vi "RT_stagectrl_readIFO_Oct.vi"() -> ()   [LabVIEW 2019]
uses:
  <vilib>/Platform/TimedLoop/XDataNode/timing_clust.ctl
  <vilib>/Platform/TimedLoop/XDataNode/nitl_modes.ctl
  <vilib>/Platform/TimedLoop/XDataNode/wakeup.ctl
  <vilib>/Analysis/baseanly.llb/Mean (DBL).vi
  <vilib>/FPGAPlugInAG/myRIO-1900/niLvFpga_Open_myRIO-1900.vi
  <vilib>/rvi/interface/common/dynamic/niFpgaDynamicAddResources.vi
  <vilib>/Utility/error.llb/Error Cluster From Error Code.vi
  <vilib>/rvi/errors/niLvFpgaAdjustHostInterfaceError.vi
  <vilib>/FPGAPlugInAG/Dynamic/niLvFpga_Close_Dynamic.vi
  <vilib>/rvi/interface/nirviOpenFPGA/nirviOpenFPGA.xnode
  FPGA Bitfiles/studentchallenge_FPGATarget_FPGA1RADC1WDAC2A_GeAN6BgpSew.lvbitx
  <vilib>/rvi/interface/nirviReadWriteControl/nirviReadWriteControl.xnode
  <vilib>/platform/TimedLoop/XDataNode/XDataNode.xnode
  <vilib>/rvi/interface/nirviCloseFPGA/nirviCloseFPGA.xnode
  NiFpgaLv.dll
  <vilib>/rvi/interface/Simulation/niFpgaSimulationCallBeginRW.vi
  <vilib>/Platform/TimedLoop/XDataNode/XDNodeRunTimeDep.lvlib
  <vilib>/Analysis/NI_AALBase.lvlib
panel:
  out "Z (um)":dbl(graph)=-1075.0316368535157
  in  "Stop":bool=TRUE
  in  "P":dbl=1.0
  in  "I":dbl=0.003
  in  "D":dbl
  out "Control voltage":dbl=-10.0 format="%#_3f"
  out "Encoder position (mm)":dbl=-1.05 format="%#_4f"
  out "late?":bool
  in  "Ramp ON":bool
  out "Mid-travel (mm)":dbl format="%#_3f"
  out "?":dynamicdata(graph)=[{"t0"=timestamp(2082851436.547542 s since 1904-01-01), "dt"=1.0, "Y"=[0.0]}, {"t0"=timestamp(2082851436.547623 s since 1904-01-01), "dt"=1.0, "Y"=[-1.05]}]
  in  "Stage loop time (us)":i64=2000
  in  "Velocity (mm/s)":dbl=0.3 format="%#_3g"
  in  "Ramp Vpp (mm)":dbl=2.0 format="%#_13g"
  out "Vp":dbl=1.05
  out "Vi":dbl=10.0
  out "Vd":dbl
  out "Lissajou":cluster{"X":dbl[], "Y":dbl[]}[](graph)
  out "?":dynamicdata(graph)=[{"t0"=timestamp(2082851436.54781 s since 1904-01-01), "dt"=1.0, "Y"=[2.36669921875]}, {"t0"=timestamp(2082851436.547639 s since 1904-01-01), "dt"=1.0, "Y"=[2.148193359375]}]
  in  "IFO plot loop time (us)":i64=1000
  out "late?":bool
  out "FWD limit flag":bool
  out "REV lim (mm)":dbl=-2.7246875 format="%#_5f"
  out "FWD lim (mm)":dbl=10.833828125 format="%#_5f"
  out "Voltage":dbl=3.5999999999999956
  out "REV limit flag":bool=TRUE
  out "Position (mm)":dbl(slide)=-2.7246875 scale=-10.0..10.0
  out "Vfwd":dbl=0.2499999999999999
  out "Vrev":dbl=-3.5999999999999956
  out "ENC0":i32=70
  out "Enc res (mm)":dbl=7.8125e-05
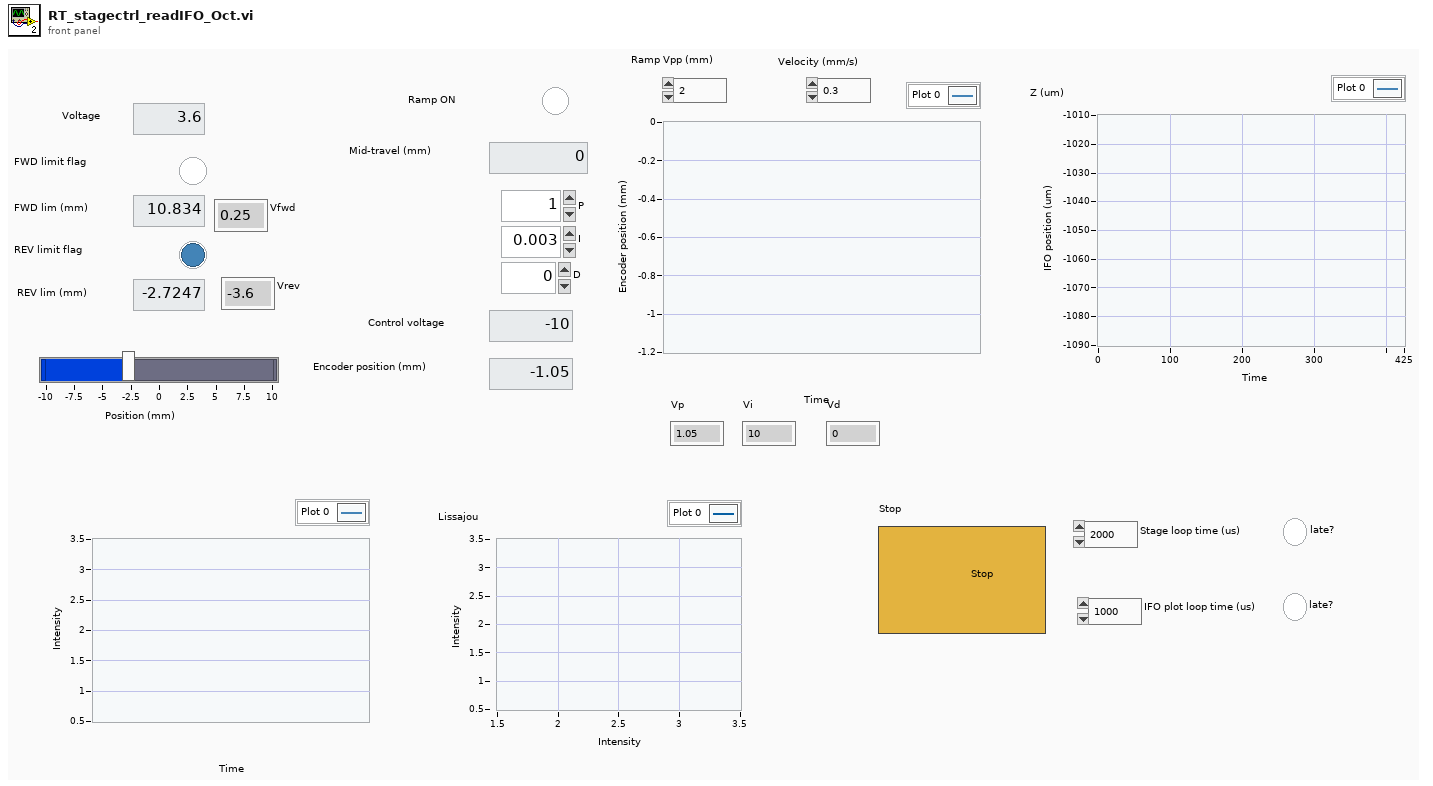
[diagram p1: front panel]
types:
  T1 = typedef "XDNodeRunTimeDep.lvlib/timing_clust.ctl" = cluster{"Expected End [f-1]":u64, "Actual End [f-1]":u64, "Finished Late? [f-1]":bool, "Expected End [i-1]":u64, "Actual End [i-1]":u64, "Finished Late? [i-1]":bool, "Expected Start [i]":u64, "Actual Start [i]":u64, "Expected Start [f]":u64, "Actual Start [f]":u64, "Source Name":string, "Structure Name":string, "Period":i64, "Deadline":i64, "Offset":i64, "Start":i64, "Priority":i32, "Timeout":i32, "Mode":T2, "Wakeup Reason":T3, "Error":errorcluster, "Source Type":string, "Secondary Source Type":string, "Global End Time":u64, "Global Start Time":u64, "Frame Duration":u64, "Iteration Duration":u64, "Assigned CPU":i32, "I/O Scan Engine Mode":u32}
  T2 = typedef "XDNodeRunTimeDep.lvlib/nitl_modes.ctl" = enum32{"No Change", "Process missed periods, maintain original phase", "Discard missed periods, maintain original phase", "Process missed periods, ignore original phase", "Discard missed periods, ignore original phase"}
  T3 = typedef "XDNodeRunTimeDep.lvlib/wakeup.ctl" = enum32{"Normal", "Aborted", "Asynchronous wakeup", "Timing source error", "Timed loop error", "Timeout"}
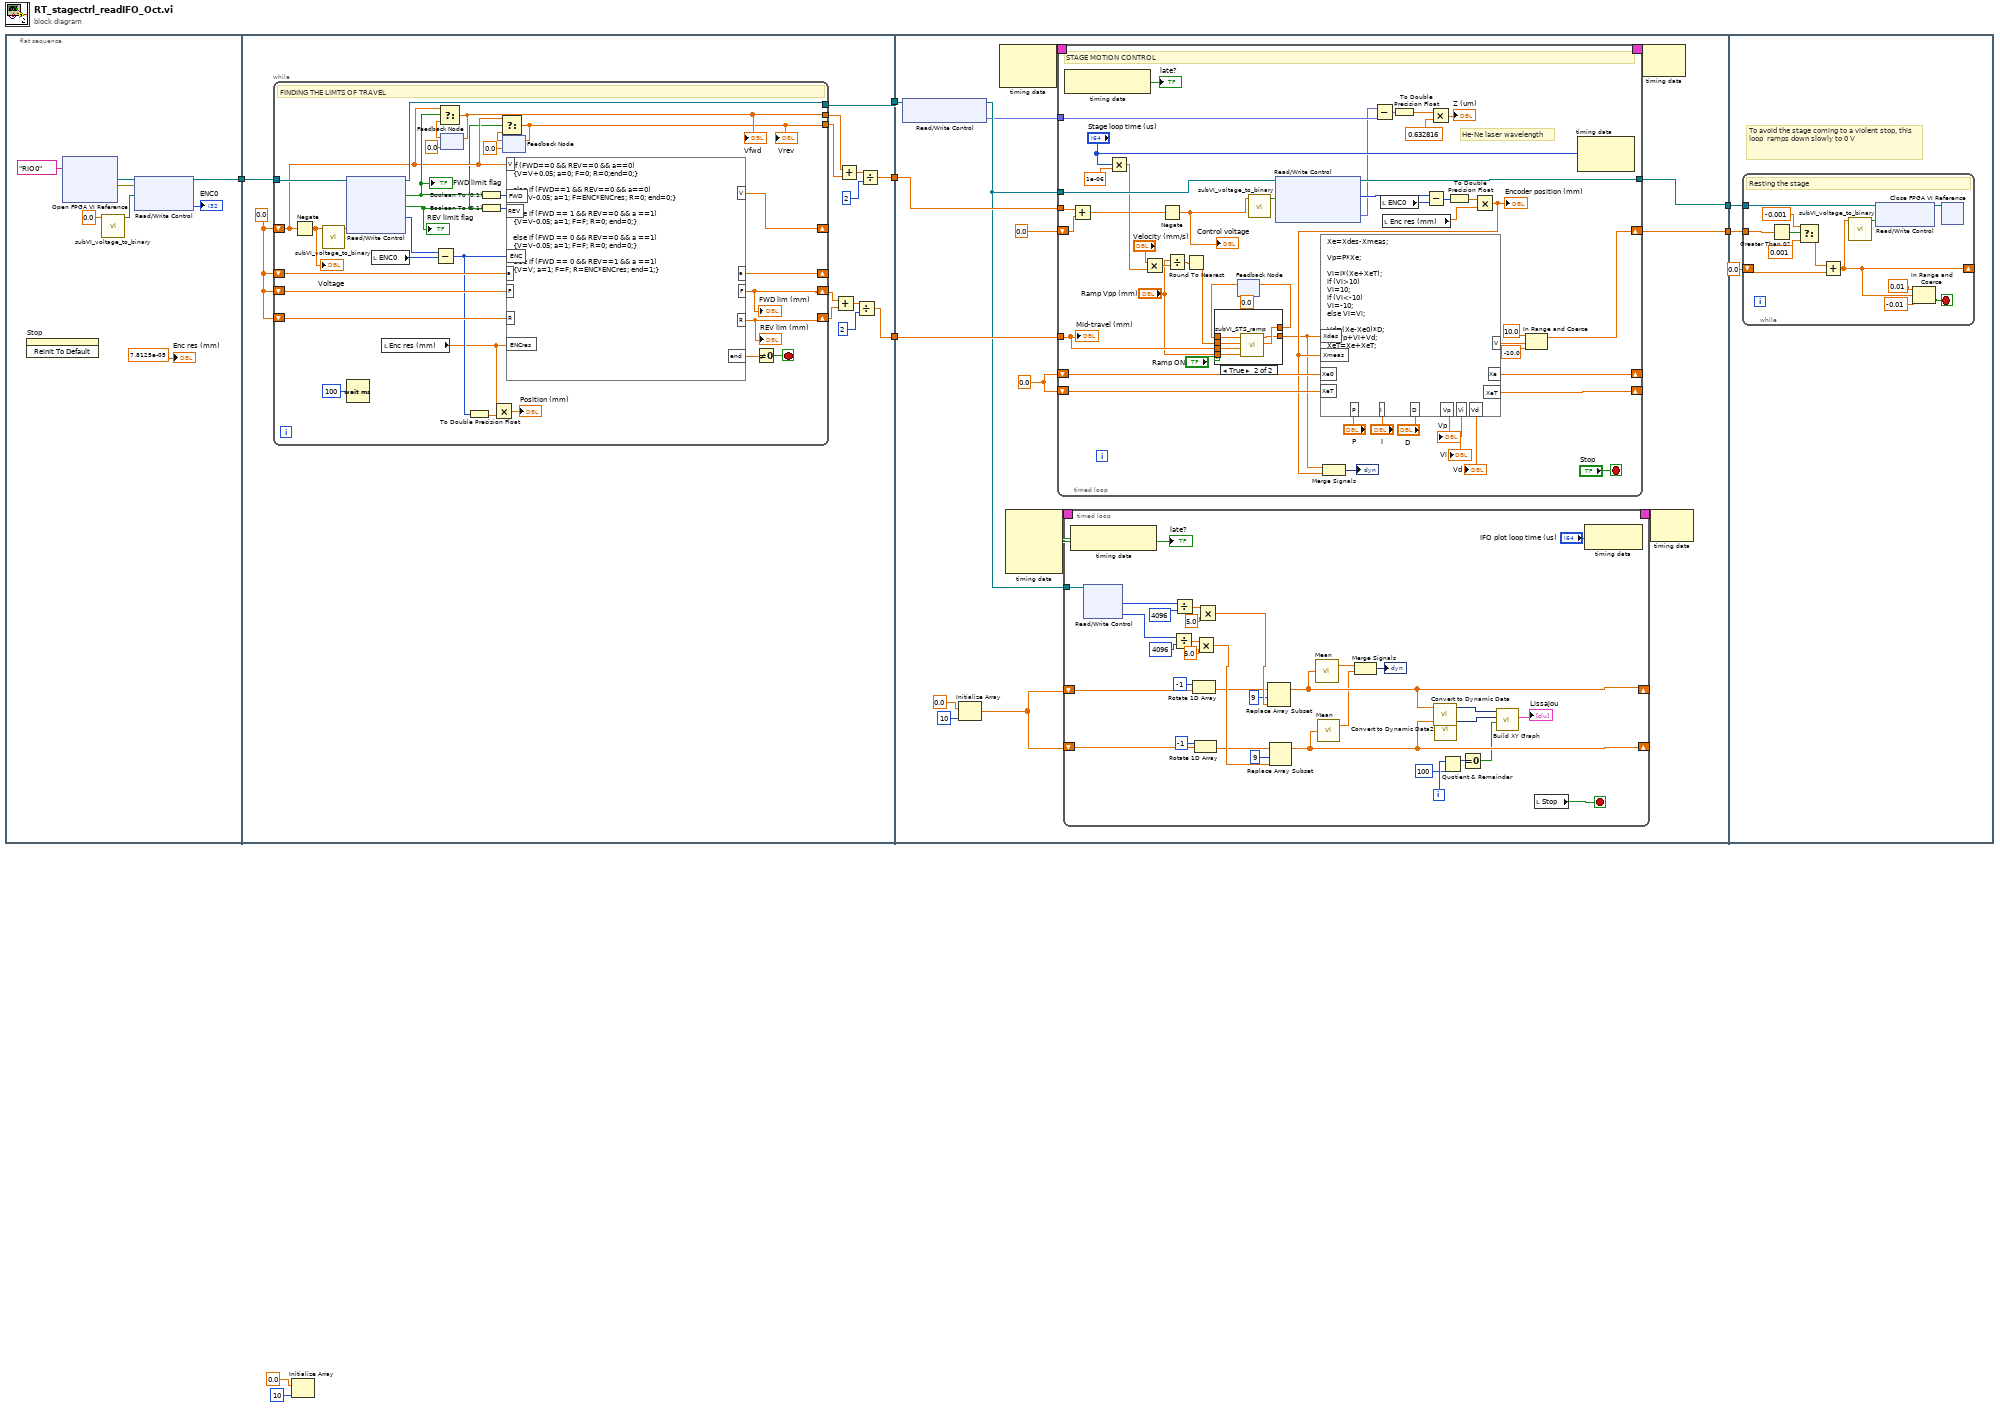
[diagram p0: block diagram]
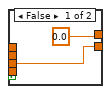
[diagram p2: hidden frame]
diagram:
  n1 = flat-sequence {
    tunnel: [w16] -> w8
    tunnel: w8 -> [w27]
    tunnel: [w29] -> w7
    tunnel: [w17] -> w6
    tunnel: [w28] -> w5
    tunnel: [w62] -> w4
    tunnel: w7 -> [w74]
    tunnel: w6 -> [w64]
    tunnel: [w73] -> w3
    tunnel: w5 -> [w65]
    tunnel: w4 -> [w185]
    tunnel: w3 -> [w184]
    frame #0 {
      n2 = invoke on="Stop" class="Bool (strict)" method="Reinit To Default"() -> ()  [unwired: 3 in, 3 out]
      n3 = xnode "Open FPGA VI Reference"("resource name"=tag "RIO0") -> ("FPGA VI Reference Out"=w9:refnum<k20>, "error out"=w14:errorcluster)  [unwired: 1 in]
      n4 = call "subVI_voltage_to_binary.vi"("voltage"=0.0) -> ("binary"=w12:bool[])  [unwired: 10 in]
      n5 = xnode "Read/Write Control"("FPGA VI Reference In"=w9, "error in"=w14, "DAC 1 write"=w12) -> ("FPGA VI Reference Out"=w16:refnum<k20>, "Encoder A"=→"ENC0":i32)  [unwired: 1 out]
      "Enc res (mm)" <- 7.8125e-05 ("y")
    }
    frame #1 {
      w22 = 0.0 ("V")
      n6 = while {
        shift-right: [w44] -> _
        shift-left: w22 -> [w33]
        shift-right: [w60] -> _
        shift-left: w22 -> [w59]
        shift-right: [w45] -> w24
        shift-left: w22 -> [w53]
        shift-right: [w46] -> w23
        shift-left: w22 -> [w52]
        tunnel: w27 -> [w50]
        tunnel: [w48] -> w17
        tunnel: [w31] -> w20
        tunnel: [w30] -> w19
        stop <- w55 stop-if-true
        # "FINDING THE LIMTS OF TRAVEL"
        n7 = Negate(x=w33) -> (-x=w39:dbl)
        "Voltage" <- w39
        n8 = call "subVI_voltage_to_binary.vi"("voltage"=w39) -> ("binary"=w51:bool[])  [unwired: 10 in]
        n9 = xnode "Read/Write Control"("FPGA VI Reference In"=w50, "DAC 1 write"=w51) -> ("FPGA VI Reference Out"=w48:refnum<k20>, "YFWD"=w38:bool, "YREV"=w32:bool, "Encoder A"=w54:i32)  [unwired: 1 in, 1 out]
        "FWD limit flag" <- w38
        "REV limit flag" <- w32
        n10 = Wait (ms)(milliseconds to wait=u32 100) -> ()  [unwired: 1 out]
        n11 = local read "ENC0"() -> (w49:i32)
        n12 = local read "Enc res (mm)"() -> (w41:dbl)
        n13 = Subtract(x=w54, y=w49) -> (x-y=w43:i32)
        n14 = feedback #1(0.0 ("V")) -> (w37:dbl)
        n15 = Select(t=w33, s=w38, f=w37) -> (s? t:f=w31:dbl)
        "Vfwd" <- w31
        n16 = feedback-in #1(w31) -> ()
        n17 = To Double Precision Float(number=w43) -> (double precision float=w40:dbl)
        n18 = Boolean To (0,1)(Boolean=w38) -> (0, 1=w58:i16)
        n19 = Boolean To (0,1)(Boolean=w32) -> (0, 1=w57:i16)
        n20 = Multiply(x=w41, y=w40) -> (x*y=→"Position (mm)":dbl)
        n21 = feedback #2(0.0 ("V")) -> (w35:dbl)
        n22 = Select(t=w33, s=w32, f=w35) -> (s? t:f=w30:dbl)
        "Vrev" <- w30
        n23 = feedback-in #2(w30) -> ()
        n24 = formula code="if (FWD==0 && REV==0 && a==0)\n{V=V+0.05; a=0; F=0; R=0;end=0;}\n\nelse if (FWD==1 && REV==0 && a==0)\n{V=V-0.05; a=1; F=ENC*ENCres; R=0; end=0;}\n\nelse if (FWD == 1 && REV==0 && a ==1)\n{V=V-0.05; a=1; F=F; R=0; end=0;}\n\nelse if (FWD == 0 && REV==0 && a ==1)\n{V=V-0.05; a=1; F=F; R=0; end=0;}\n\nelse if (FWD == 0 && REV==1 && a ==1)\n{V=V; a=1; F=F; R=ENC*ENCres; end=1;}"("FWD"=w58, "REV"=w57, "a"=w59, "ENC"=w43, "F"=w53, "R"=w52, "V"=w33, "ENCres"=w41) -> ("V"=w44:dbl, "a"=w60:dbl, "end"=w56:dbl, "F"=w45:dbl, "R"=w46:dbl)
        "REV lim (mm)" <- w46
        "FWD lim (mm)" <- w45
        n25 = Not Equal To 0?(x=w56) -> (x != 0?=w55:bool)
      }
      n26 = Add(x=w24, y=w23) -> (x+y=w26:dbl)
      n27 = Add(x=w20, y=w19) -> (x+y=w18:dbl)
      n28 = Divide(x=w26, y=2) -> (x/y=w29:dbl)
      n29 = Divide(x=w18, y=2) -> (x/y=w28:dbl)
    }
    frame #2 {
      w67 = 0.0 ("Xe")
      n30 = xnode "Read/Write Control"("FPGA VI Reference In"=w64) -> ("FPGA VI Reference Out"=w63:refnum<k20>, "unwrapped phase"=w61:fxp<+/-,47,33>)  [unwired: 1 in, 1 out]
      n31 = Initialize Array(0.0 ("element"), 10 ("dimension size")) -> (w68:dbl[])
      n32 = node-c288() -> (w76:T1)  [unwired: 2 in]
      n33 = node-c288() -> (w72:T1)  [unwired: 4 in]
      n34 = timed-loop {
        timing: w76 -> [_]
        timing-out: [_] -> w75
        tunnel: [w163] -> w62
        tunnel: w74 -> [w133]
        shift-right: [w148] -> w73
        shift-left: 0.0 ("upper limit") -> [w127]
        tunnel: w63 -> [w161]
        shift-right: [w156] -> _
        shift-left: w67 -> [w155]
        shift-right: [w154] -> _
        shift-left: w67 -> [w153]
        tunnel: w65 -> [w126]
        tunnel: w61 -> [w120]
        stop <- "Stop" stop-if-true
        # "He-Ne laser wavelength"
        # "STAGE MOTION CONTROL"
        n35 = node-c288() -> (→"late?":bool)  [unwired: 1 in]
        n36 = Add(x=w126, y=w127) -> (x+y=w124:dbl)
        n37 = Multiply(x="Stage loop time (us)", y=1e-06) -> (x*y=w141:dbl)
        n38 = Multiply(x="Velocity (mm/s)", y=w141) -> (x*y=w144:dbl)
        n39 = Negate(x=w124) -> (-x=w125:dbl)
        "Control voltage" <- w125
        n40 = Divide(x="Ramp Vpp (mm)", y=w144) -> (x/y=w139:dbl)
        n41 = Round To Nearest(number=w139) -> (nearest integer value=w134:dbl)
        n42 = feedback #3(0.0 ("n1")) -> (w136:dbl)
        n43 = case shown="True" "Ramp ON" {
          tunnel: w136 -> [_ w175]
          tunnel: [0.0 ("n1") w174] -> w135
          tunnel: w134 -> [_ w173]
          tunnel: w133 -> [w169 w172]
          tunnel: [w169 w171] -> w131
          tunnel: "Ramp Vpp (mm)" -> [_ w170]
          frame False {
          }
          frame True {
            n44 = call "subVI_STS_ramp.vi"("Ramp Vpp"=w170, "Ramp offset"=w172, "Ramp datapoints"=w173, "n"=w175) -> ("n1"=w174:dbl, "Ramp out"=w171:dbl)  [unwired: 6 in]
          }
        }
        n45 = feedback-in #3(w135) -> ()
        n46 = call "subVI_voltage_to_binary.vi"("voltage"=w125) -> ("binary"=w164:bool[])  [unwired: 10 in]
        n47 = xnode "Read/Write Control"("FPGA VI Reference In"=w161, "DAC 1 write"=w164) -> ("FPGA VI Reference Out"=w163:refnum<k20>, "Encoder A"=w165:i32, "unwrapped phase"=w119:fxp<+/-,47,33>)  [unwired: 1 in, 1 out]
        n48 = Subtract(x=w119, y=w120) -> (x-y=w121:fxp<+/-,48,34>)
        n49 = local read "ENC0"() -> (w162:i32)
        n50 = local read "Enc res (mm)"() -> (w145:dbl)
        n51 = To Double Precision Float(number=w121) -> (double precision float=w123:dbl)
        n52 = Subtract(x=w165, y=w162) -> (x-y=w166:i32)
        n53 = Multiply(x=w123, y=0.632816) -> (x*y=→"Z (um)":dbl)
        n54 = To Double Precision Float(number=w166) -> (double precision float=w167:dbl)
        n55 = Multiply(x=w167, y=w145) -> (x*y=w146:dbl)
        "Encoder position (mm)" <- w146
        n56 = formula code="Xe=Xdes-Xmeas;\n\nVp=P*Xe;\n\nVi=I*(Xe+XeT);\nif (Vi>10)\nVi=10;\nif (Vi<-10)\nVi=-10;\nelse Vi=Vi;\n\nVd=(Xe-Xe0)*D;\nV=Vp+Vi+Vd;\nXeT=Xe+XeT;"("Xdes"=w131, "Xmeas"=w146, "Xe0"=w155, "XeT"=w153, "P"="P", "I"="I", "D"="D") -> ("Xe"=w156:dbl, "V"=w157:dbl, "XeT"=w154:dbl, "Vp"=→"Vp":dbl, "Vi"=→"Vi":dbl, "Vd"=→"Vd":dbl)
        n57 = Merge Signals(w131, w146) -> (→"?":dynamicdata)
        n58 = In Range and Coerce(upper limit=10.0, x=w157, lower limit=-10.0) -> (coerced(x)=w148:dbl)  [unwired: 1 out]
        n59 = node-c288("Stage loop time (us)") -> ()  [unwired: 1 in, 1 out]
        "Mid-travel (mm)" <- w133
      }
      n60 = timed-loop {
        shift-right: [w108] -> _
        shift-left: w68 -> [w110]
        shift-right: [w107] -> _
        shift-left: w68 -> [w109]
        timing: w72 -> [_]
        timing-out: [_] -> w71
        tunnel: w63 -> [w104]
        i -> [w106]
        stop <- w103 stop-if-true
        n61 = node-c288() -> (→"late?":bool)  [unwired: 1 in]
        n62 = xnode "Read/Write Control"("FPGA VI Reference In"=w104) -> ("PD1"=w95:u16, "PD2"=w94:u16)  [unwired: 1 in, 2 out]
        n63 = Divide(x=w94, y=u16 4096) -> (x/y=w98:dbl)
        n64 = Divide(x=w95, y=u16 4096) -> (x/y=w100:dbl)
        n65 = Rotate 1D Array(1:w110, 2:-1 ("n")) -> (0:w90:dbl[])
        n66 = Rotate 1D Array(1:w109, 2:-1 ("n")) -> (0:w87:dbl[])
        n67 = Multiply(x=w98, y=5.0) -> (x*y=w92:dbl)
        n68 = Multiply(x=w100, y=5.0) -> (x*y=w93:dbl)
        n69 = Replace Array Subset(array=w90, new element=w93, index=9) -> (w108:dbl[])
        n70 = Replace Array Subset(array=w87, new element=w92, index=9) -> (w107:dbl[])
        n71 = call-poly <vilib>:"Mean.vi"("X"=w108) -> ("mean"=w79:dbl)  [unwired: 1 out]
        n72 = call-poly <vilib>:"Mean.vi"("X"=w107) -> ("mean"=w78:dbl)  [unwired: 1 out]
        n73 = Merge Signals(w79, w78) -> (→"?":dynamicdata)
        n74 = call "Convert to Dynamic Data"("Array"=w108) -> ("Dynamic Data Type"=w85:dynamicdata)  [unwired: 3 in]
        n75 = call "Convert to Dynamic Data2"("Array"=w107) -> ("Dynamic Data Type"=w84:dynamicdata)  [unwired: 3 in]
        n76 = Quotient & Remainder(x=w106, y=100) -> (x-y*floor(x/y)=w81:i32)  [unwired: 1 out]
        n77 = Equal To 0?(x=w81) -> (x = 0?=w82:bool)
        n78 = call "Build XY Graph"("Reset"=w82, "Y Input"=w84, "X Input"=w85) -> ("XY Graph"=→"Lissajou":cluster{"X":dbl[], "Y":dbl[]}[])  [unwired: 7 in, 1 out]
        n79 = local read "Stop"() -> (w103:bool)
        n80 = node-c288("IFO plot loop time (us)") -> ()  [unwired: 1 out]
      }
      n81 = node-c288(w75) -> ()  [unwired: 1 out]
      n82 = node-c288(w71) -> ()  [unwired: 1 out]
    }
    frame #3 {
      # "To avoid the stage coming to a violent stop, this loop  ramps down slowly to 0 V"
      n83 = while {
        tunnel: w185 -> [w196]
        tunnel: w184 -> [w187]
        shift-right: [w186] -> _
        shift-left: 0.0 -> [w191]
        stop <- w188 stop-if-true
        # "Resting the stage"
        n84 = Greater Than 0?(x=w187) -> (x > 0?=w195:bool)
        n85 = Select(t=-0.001, s=w195, f=0.001) -> (s? t:f=w192:dbl)
        n86 = Add(x=w192, y=w191) -> (x+y=w186:dbl)
        n87 = call "subVI_voltage_to_binary.vi"("voltage"=w186) -> ("binary"=w198:bool[])  [unwired: 10 in]
        n88 = xnode "Read/Write Control"("FPGA VI Reference In"=w196, "DAC 1 write"=w198) -> ("FPGA VI Reference Out"=w197:refnum<k20>)  [unwired: 1 in, 1 out]
        n89 = In Range and Coerce(upper limit=0.01, x=w186, lower limit=-0.01) -> (In Range?=w188:bool)  [unwired: 1 out]
        n90 = xnode "Close FPGA VI Reference"("FPGA VI Reference In"=w197) -> ()  [unwired: 1 in, 1 out]
      }
    }
  }
  n91 = Initialize Array(0.0 ("element"), 10 ("dimension size")) -> ()  [unwired: 1 out]
